vi "getWidth.vi"(0 "HGF_ImaqDx in":refnum<class "HGF_ImaqDx.lvclass">, 5 "error in (no error)":errorcluster) -> (14 "HGF_ImaqDx out":refnum<class "HGF_ImaqDx.lvclass">, 17 "Width":i32, 19 "error out":errorcluster)   [LabVIEW 2014, in "HGF_IMAQ.lvlib" / "HGF_ImaqDx.lvclass"]
doc: "Returns the width of the image taken by the camera."
uses:
  HGF_ImaqDx.lvclass
  <resource>/objmgr/imaqdx.rc
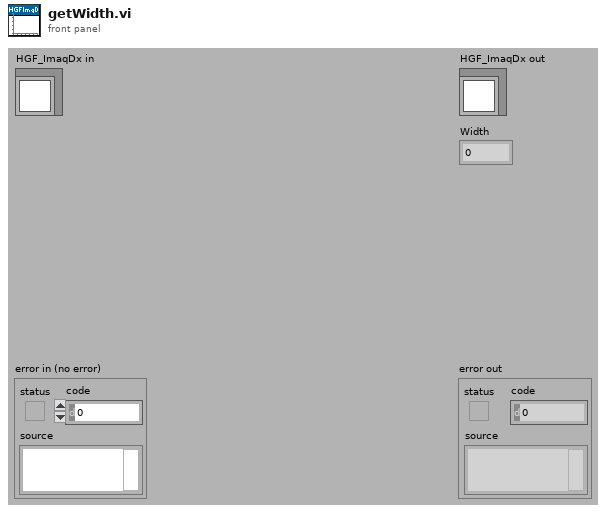
[diagram p1: front panel]
types:
  T1 = typedef "IMAQdx.ctl" = refnum<k21>
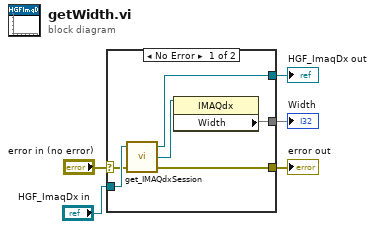
[diagram p0: block diagram]
diagram:
  n1 = case shown="No Error" "error in (no error)" {
    selector: "error in (no error)" -> [w6 w13]
    tunnel: "HGF_ImaqDx in" -> [w11 w12]
    tunnel: [w9 w12] -> w4
    tunnel: [w8 w13] -> w3
    tunnel: [w7 _] -> w2
    frame No Error {
      n2 = call "get_IMAQdxSession.vi"("error in (no error)"=w6, "HGF_ImaqDx in"=w11) -> ("error out"=w8:errorcluster, "IMAQdx Session"=w10:T1, "HGF_ImaqDx out"=w9:refnum<class "HGF_ImaqDx.lvclass">)  [unwired: 1 in]
      n3 = property class="IMAQdx"(reference=w10) -> ("Width"=w7)  [unwired: 1 in, 2 out]
    }
    frame Error {
    }
  }
  "error out" <- w3
  "HGF_ImaqDx out" <- w4
  "Width" <- w2
